vi "Controller FA File Management Loop.vi"(7 "Sync Objects":T1, 8 "error in (no error)":errorcluster, 11 "FOFB Configuration":T5={"FOFB Parameters"={"Network"={"FOFB Controller IP"="", "LNLS Control Network IP"="", "LNLS Control Network Power Supplies TCP Port"=0, "LNLS Control Network FOFB Configuration TCP Port"=0, "Data Server TCP Port"=0, "Monitoring Data TCP Port"=0, "Configuration GUI TCP Port"=0, "TCP Listening Timeout"=0}, "Fast Acquisition"={"Acquisition Period"=0, "Data Buffer Size"=0}, "Response Matrix Measurement"={"Step Amplitude"=0.0, "Time Between Steps"=0, "Step Duration"=0, "Number of Averages"=0}, "Correction Algorithm"={"Correction Period"=0, "Reference Orbit Path"=path "", "Response Matrix Path"=path "", "Correction Matrix Path"=path "", "Horizontal Correction Factor"=0.0, "Vertical Correction Factor"=0.0, "Beam Current FOFB Threshold"=0.0, "Decouple H-V"=FALSE}, "Acquisition Network"=[], "Actuation Network"=[]}, "Number of Acquisition Chassis"=0, "Number of Actuation Chassis"=0, "Number of BPM Readings"=0, "BPM Reading Names"=[], "Selected BPM Readings"=[0, 1, 2, 3, 4, 5, 6, 7, 8, 9, 10, 11, 12, 13, 14, 15, 16, 17, 18, 19, 20, 21, 22, 23, 24, 25, 26, 27, 28, 29, 30, 31, 32, 33, 34, 35, 36, 37, 38, 39, 40, 41, 42, 43, 44, 45, 46, 47, 48, 49], "Number of Correctors"=0, "Corrector Names"=[], "Selected Correctors"=[0, 1, 2, 3, 4, 5, 6, 7, 8, 9, 10, 11, 12, 13, 14, 15, 16, 17, 18, 19, 20, 21, 22, 23, 24, 25, 26, 27, 28, 29, 30, 31, 32, 33, 34, 35, 36, 37, 38, 39, 40, 41, 42, 43, 44, 45, 46, 47, 48, 49], "Reference Orbit"=[], "Response Matrix"=[], "Correction Matrix"=[], "Acquisition Chassis Names"=[], "Actuation Chassis Names"=[], "Acquisition Variables"=[], "Actuation Variables"=[], "PS Matrix Mapping"=[], "Inverse PS Matrix Mapping"=[], "Response Matrix Beam Energy (MeV)"=0.0, "PID Parameters"=[], "BPM Planes"=[], "Corrector Planes"=[], "RMM Step Factor"=[]}) -> (0 "error out":errorcluster)   [LabVIEW 2011, in "Controller VIs.lvlib"]
uses:
  Controller VIs.lvlib
  Types Definitions/Type FOFB Configuration.ctl
  Types Definitions/Type FOFB Parameters.ctl
  Types Definitions/Type Network Configuration.ctl
  Types Definitions/Type FA Configuration.ctl
  Types Definitions/Type Response Matrix Measurement Configuration.ctl
  Types Definitions/Type Correction Algorithm Configuration.ctl
  Types Definitions/Type Acquisition Network Configuration.ctl
  Types Definitions/Type Actuation Network Configuration.ctl
  Types Definitions/Type PID Parameters.ctl
  Types Definitions/Type Synchronization Objects.ctl
  Types Definitions/Type Blocking Synchronization Objects.ctl
  Types Definitions/Type FA Request Parameters.ctl
  Types Definitions/Type BPM and PS select cluster.ctl
  Types Definitions/Type FA File Parameters.ctl
  Types Definitions/Type Monitoring Data.ctl
  Types Definitions/Type Diagnostics Data.ctl
  Types Definitions/Type CPU Loads Array.ctl
  Types Definitions/Type CPU Loads.ctl
  Types Definitions/Type Non-blocking Synchronization Objects.ctl
  Types Definitions/Type FOFB Variables.ctl
  Types Definitions/Type Actuation State.ctl
  <vilib>/Platform/TimedLoop/XDataNode/timing_clust.ctl
  <vilib>/Platform/TimedLoop/XDataNode/nitl_modes.ctl
  <vilib>/Platform/TimedLoop/XDataNode/wakeup.ctl
  <vilib>/Platform/TimedLoop/XDataNode/XDataNode.xnode
  File VIs.lvlib
  Type Definitions.lvlib
  Common VIs.lvlib
  <vilib>/Platform/TimedLoop/XDataNode/XDNodeRunTimeDep.lvlib
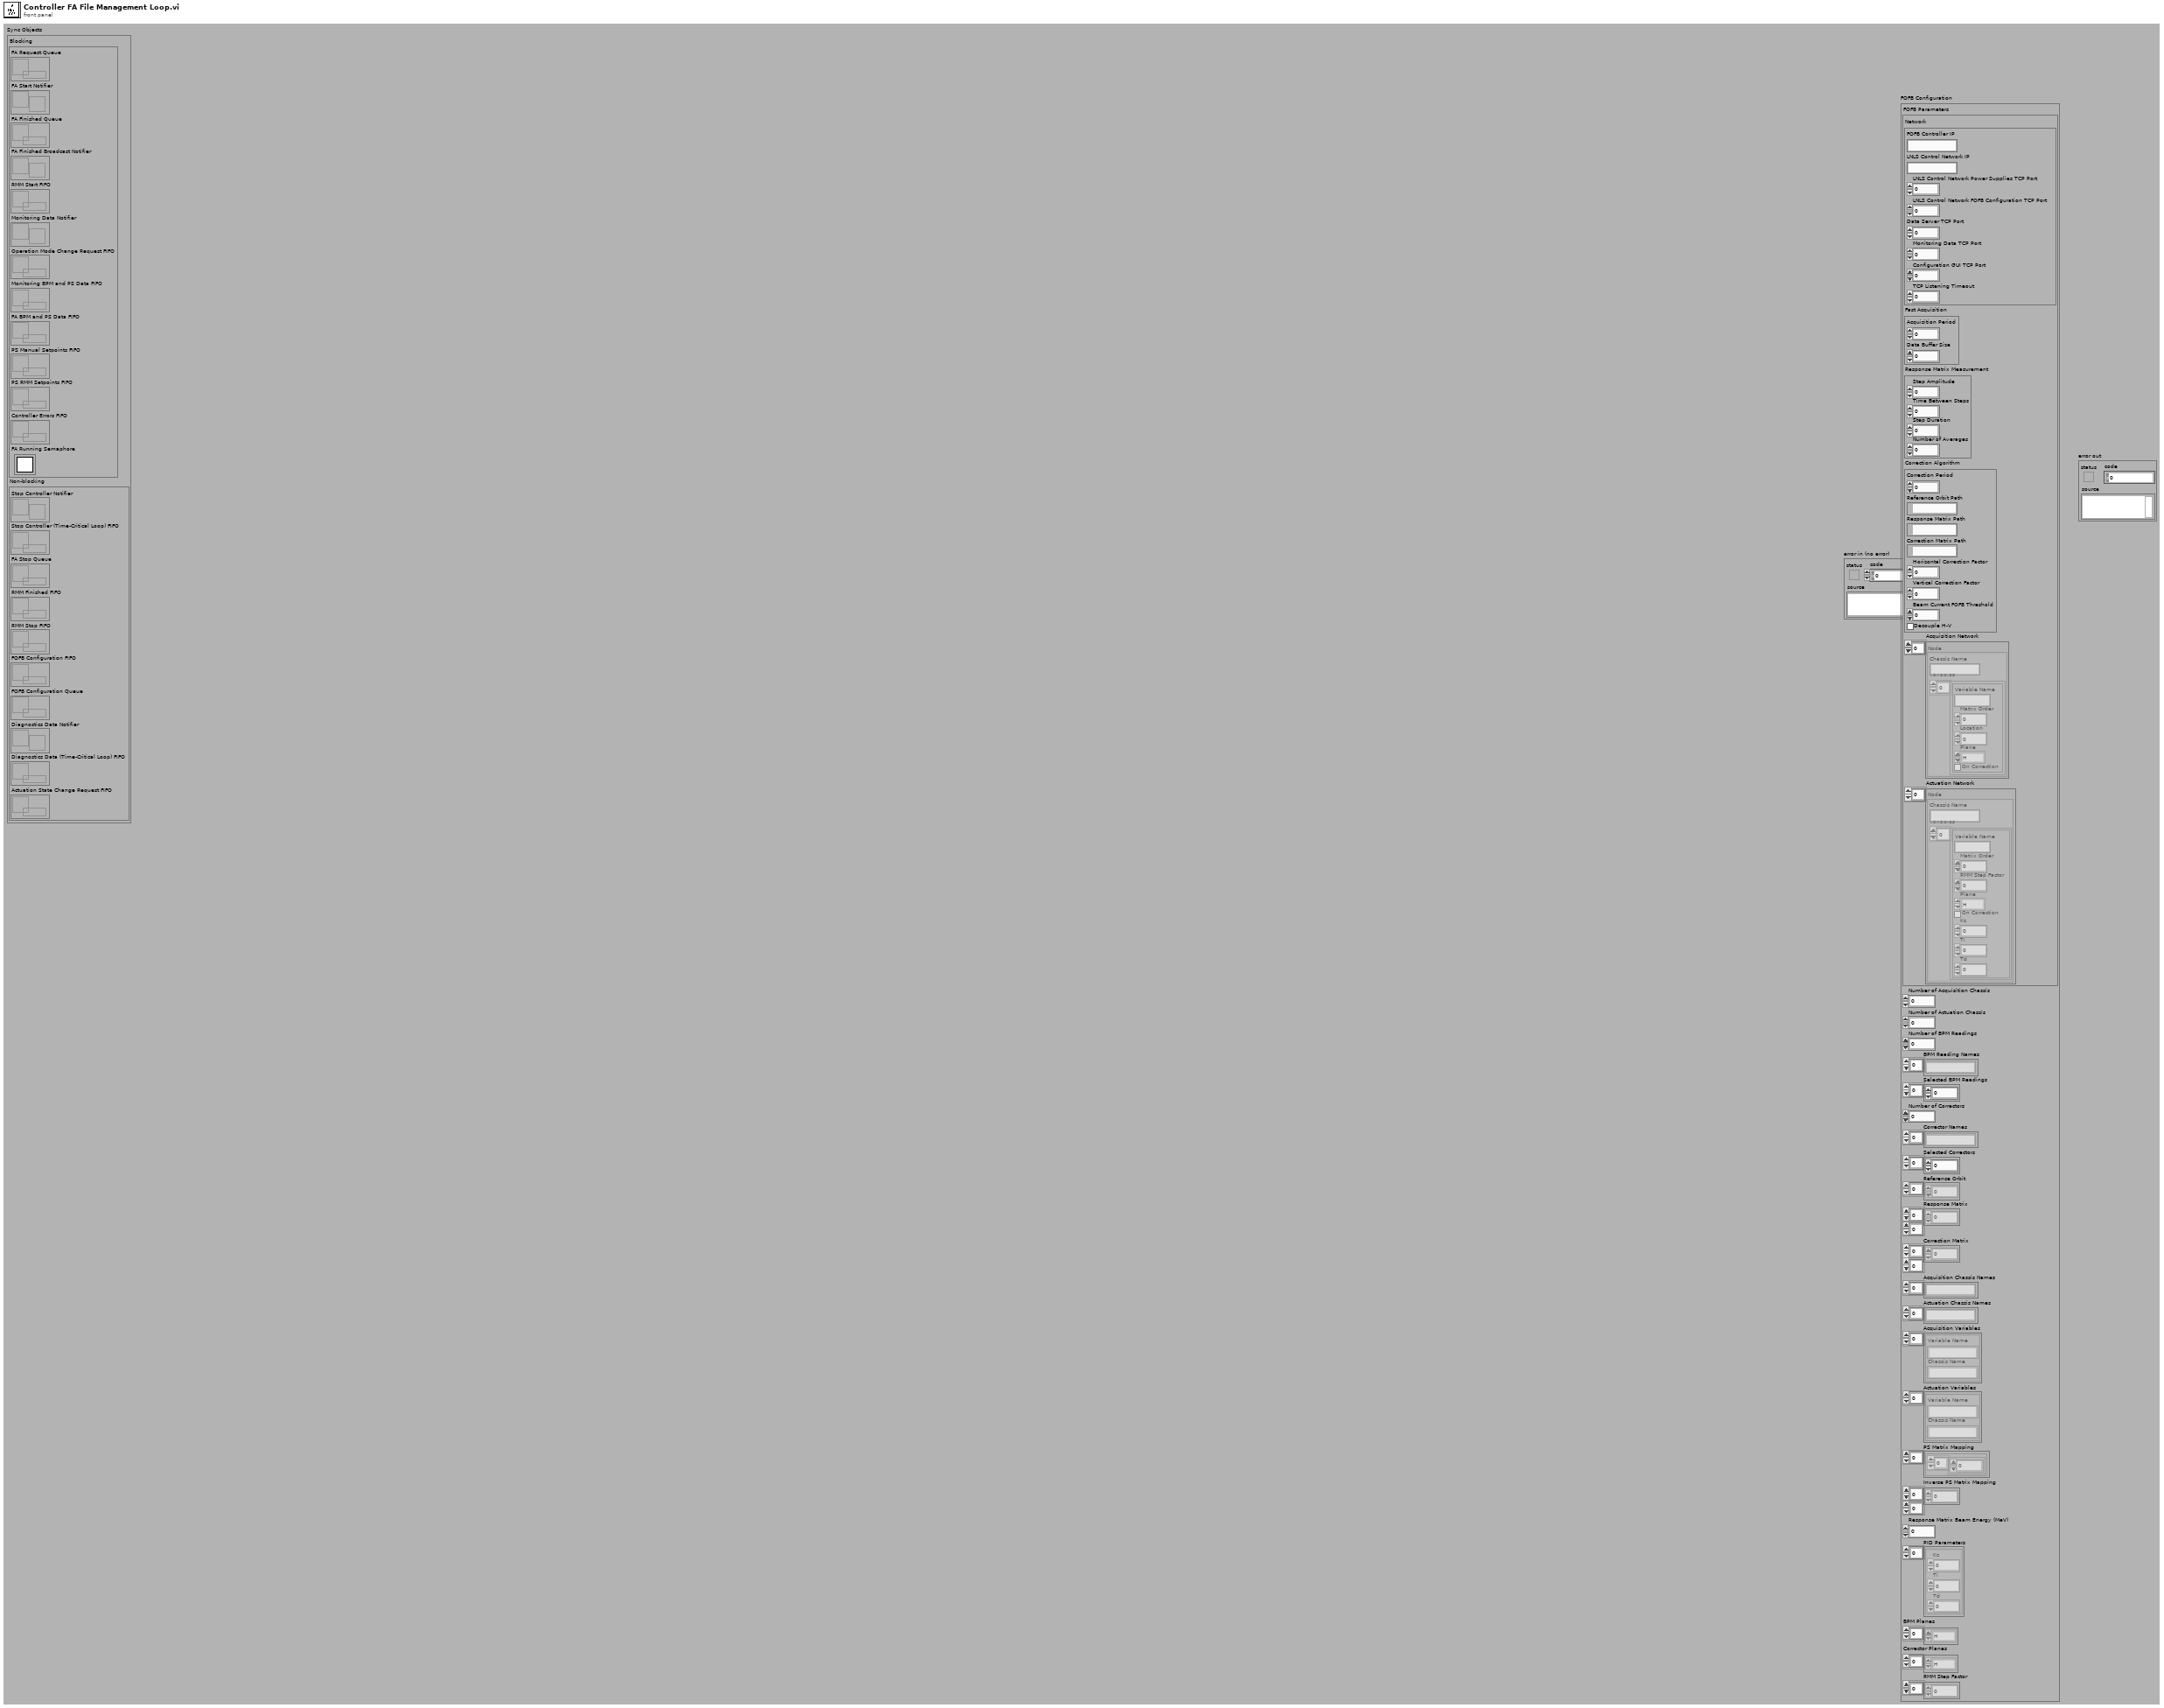
[diagram p1: front panel]
types:
  T1 = typedef "Type Definitions.lvlib/Type Synchronization Objects.ctl" = cluster{"Blocking":T2, "Non-blocking":T4}
  T2 = typedef "Type Definitions.lvlib/Type Blocking Synchronization Objects.ctl" = cluster{"FA Request Queue":refnum<queue>, "FA Start Notifier":refnum<notifier>, "FA Finished Queue":refnum<queue>, "FA Finished Broadcast Notifier":refnum<notifier>, "RMM Start FIFO":refnum<k33>, "Monitoring Data Notifier":refnum<notifier>, "Operation Mode Change Request FIFO":refnum<k33>, "Monitoring BPM and PS Data FIFO":refnum<k33>, "FA BPM and PS Data FIFO":refnum<k33>, "PS Manual Setpoints FIFO":refnum<k33>, "PS RMM Setpoints FIFO":refnum<k33>, "Controller Errors FIFO":refnum<k33>, "FA Running Semaphore":T3}
  T3 = typedef "Semaphore RefNum" = refnum<k1>
  T4 = typedef "Type Definitions.lvlib/Type Non-blocking Synchronization Objects.ctl" = cluster{"Stop Controller Notifier":refnum<notifier>, "Stop Controller (Time-Critical Loop) FIFO":refnum<k33>, "FA Stop Queue":refnum<queue>, "RMM Finished FIFO":refnum<k33>, "RMM Stop FIFO":refnum<k33>, "FOFB Configuration FIFO":refnum<k33>, "FOFB Configuration Queue":refnum<queue>, "Diagnostics Data Notifier":refnum<notifier>, "Diagnostics Data (Time-Critical Loop) FIFO":refnum<k33>, "Actuation State Change Request FIFO":refnum<k33>}
  T5 = typedef "Type Definitions.lvlib/Type FOFB Configuration.ctl" = cluster{"FOFB Parameters":T6, "Number of Acquisition Chassis":i32, "Number of Actuation Chassis":i32, "Number of BPM Readings":i32, "BPM Reading Names":string[], "Selected BPM Readings":u32[], "Number of Correctors":i32, "Corrector Names":string[], "Selected Correctors":u32[], "Reference Orbit":dbl[], "Response Matrix":dbl[][], "Correction Matrix":dbl[][], "Acquisition Chassis Names":string[], "Actuation Chassis Names":string[], "Acquisition Variables":cluster{"Variable Name":string, "Chassis Name":string}[], "Actuation Variables":cluster{"Variable Name":string, "Chassis Name":string}[], "PS Matrix Mapping":cluster{u32[]}[], "Inverse PS Matrix Mapping":u32[][], "Response Matrix Beam Energy (MeV)":dbl, "PID Parameters":T13[], "BPM Planes":enum8{"H", "V"}[], "Corrector Planes":enum8{"H", "V"}[], "RMM Step Factor":dbl[]}
  T6 = typedef "Type Definitions.lvlib/Type FOFB Parameters.ctl" = cluster{"Network":T7, "Fast Acquisition":T8, "Response Matrix Measurement":T9, "Correction Algorithm":T10, "Acquisition Network":T11, "Actuation Network":T12}
  T7 = typedef "Type Definitions.lvlib/Type Network Configuration.ctl" = cluster{"FOFB Controller IP":string, "LNLS Control Network IP":string, "LNLS Control Network Power Supplies TCP Port":u16, "LNLS Control Network FOFB Configuration TCP Port":u16, "Data Server TCP Port":u16, "Monitoring Data TCP Port":u16, "Configuration GUI TCP Port":u16, "TCP Listening Timeout":i32}
  T8 = typedef "Type Definitions.lvlib/Type FA Configuration.ctl" = cluster{"Acquisition Period":u32, "Data Buffer Size":u32}
  T9 = typedef "Type Definitions.lvlib/Type Response Matrix Measurement Configuration.ctl" = cluster{"Step Amplitude":dbl, "Time Between Steps":u32, "Step Duration":u32, "Number of Averages":u32}
  T10 = typedef "Type Definitions.lvlib/Type Correction Algorithm Configuration.ctl" = cluster{"Correction Period":u32, "Reference Orbit Path":path, "Response Matrix Path":path, "Correction Matrix Path":path, "Horizontal Correction Factor":dbl, "Vertical Correction Factor":dbl, "Beam Current FOFB Threshold":dbl, "Decouple H-V":bool}
  T11 = typedef "Type Definitions.lvlib/Type Acquisition Network Configuration.ctl" = cluster{"Chassis Name":string, "Variables":cluster{"Variable Name":string, "Matrix Order":u32, "Location":dbl, "Plane":enum8{"H", "V"}, "On Correction":bool}[]}[]
  T12 = typedef "Type Definitions.lvlib/Type Actuation Network Configuration.ctl" = cluster{"Chassis Name":string, "Variables":cluster{"Variable Name":string, "Matrix Order":u32, "RMM Step Factor":dbl, "Plane":enum8{"H", "V"}, "On Correction":bool, "Kc":dbl, "Ti":dbl, "Td":dbl}[]}[]
  T13 = typedef "Type Definitions.lvlib/Type PID Parameters.ctl" = cluster{"Kc":fxp<+/-,16,8>, "Ti":fxp<+/-,16,8>, "Td":fxp<+/-,16,8>}
  T14 = typedef "XDNodeRunTimeDep.lvlib/timing_clust.ctl" = cluster{"Expected End [f-1]":u64, "Actual End [f-1]":u64, "Finished Late? [f-1]":bool, "Expected End [i-1]":u64, "Actual End [i-1]":u64, "Finished Late? [i-1]":bool, "Expected Start [i]":u64, "Actual Start [i]":u64, "Expected Start [f]":u64, "Actual Start [f]":u64, "Source Name":string, "Structure Name":string, "Period":i64, "Deadline":i64, "Offset":i64, "Start":i64, "Priority":i32, "Timeout":i32, "Mode":T15, "Wakeup Reason":T16, "Error":errorcluster, "Source Type":string, "Secondary Source Type":string, "Global End Time":u64, "Global Start Time":u64, "Frame Duration":u64, "Iteration Duration":u64, "Assigned CPU":i32, "I/O Scan Engine Mode":u32}
  T15 = typedef "XDNodeRunTimeDep.lvlib/nitl_modes.ctl" = enum32{"No Change", "Process missed periods, maintain original phase", "Discard missed periods, maintain original phase", "Process missed periods, ignore original phase", "Discard missed periods, ignore original phase"}
  T16 = typedef "XDNodeRunTimeDep.lvlib/wakeup.ctl" = enum32{"Normal", "Aborted", "Asynchronous wakeup", "Timing source error", "Timed loop error", "Timeout"}
  T17 = typedef "Type Definitions.lvlib/Type FA File Parameters.ctl" = cluster{"FA Parameters":T18, "File Reference":refnum<file>}
  T18 = typedef "Type Definitions.lvlib/Type FA Request Parameters.ctl" = cluster{"Number of Samples":u32, "BPM and PS Selection":T19, "Filename":string}
  T19 = typedef "Type Definitions.lvlib/Type BPM and PS select cluster.ctl" = cluster{"BPM index array":u32[], "PS index array ":u32[]}
  T20 = enum16{"open", "replace", "create", "open or create", "replace or create", "replace or create with confirmation"}
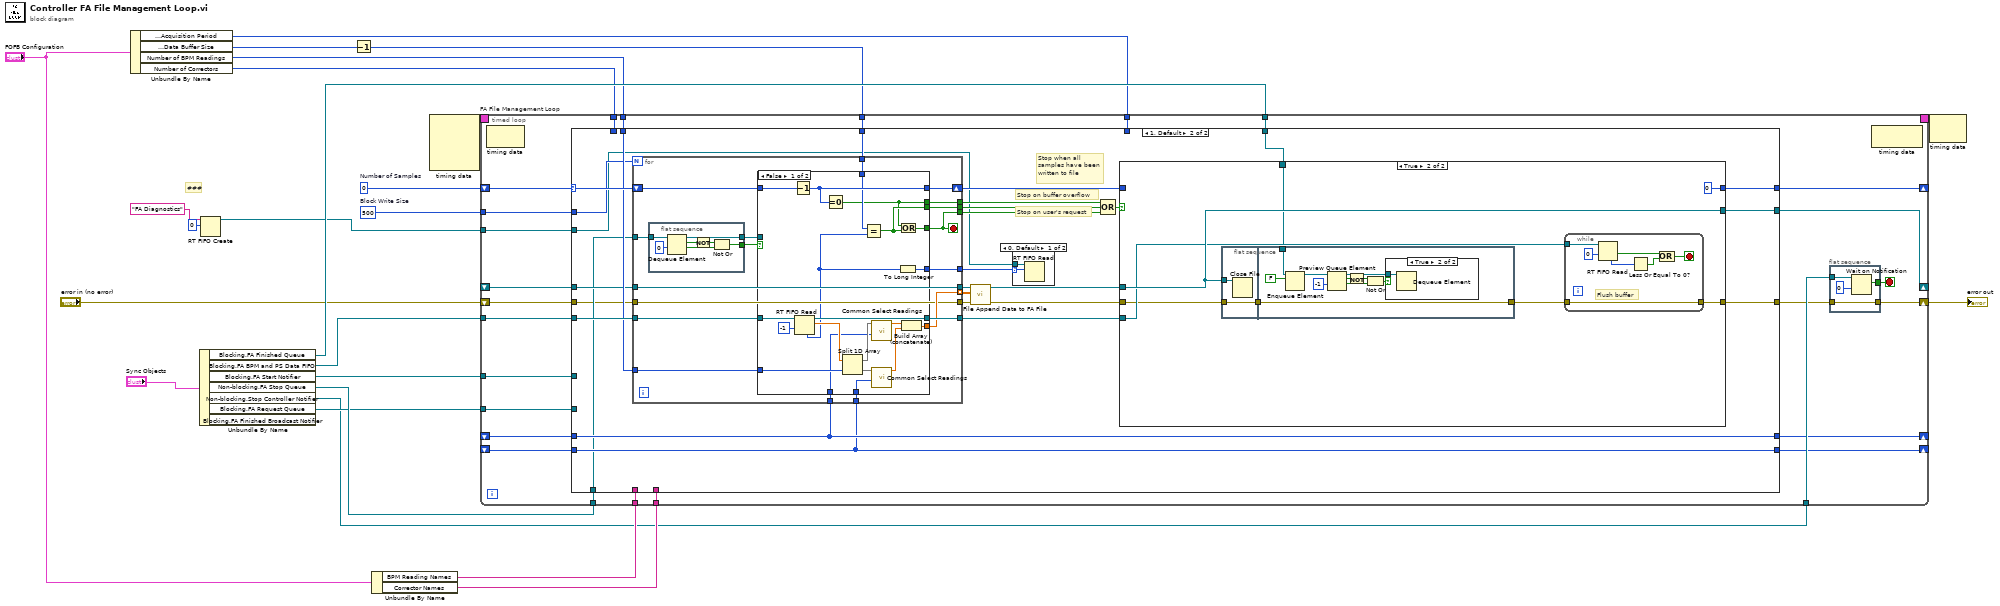
[diagram p0: block diagram]
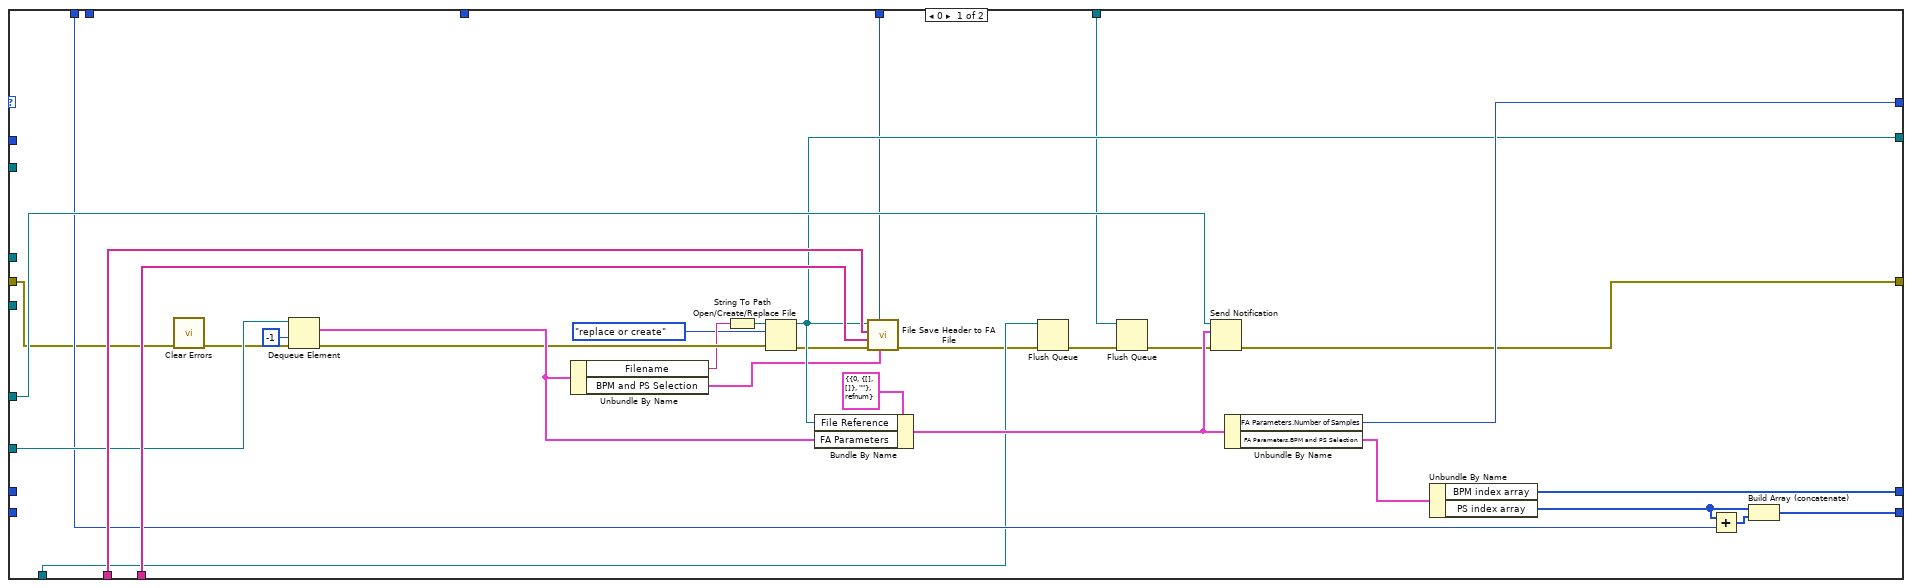
[diagram p2: hidden frame]
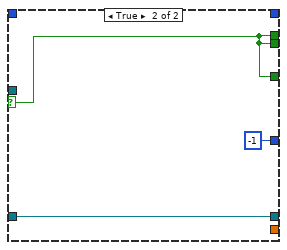
[diagram p4: hidden frame]
diagram:
  w7 = 500  # Block Write Size
  w22 = u32 0  # Number of Samples
  # "###"
  n1 = Unbundle By Name("FOFB Configuration") -> ("FOFB Parameters.Fast Acquisition.Acquisition Period"=w6:u32, "FOFB Parameters.Fast Acquisition.Data Buffer Size"=w20:u32, "Number of BPM Readings"=w9:i32, "Number of Correctors"=w8:i32)
  n2 = Unbundle By Name("Sync Objects") -> ("Blocking.FA Finished Queue"=w21:refnum<queue>, "Blocking.FA BPM and PS Data FIFO"=w23:refnum<k33>, "Blocking.FA Start Notifier"=w13:refnum<notifier>, "Non-blocking.FA Stop Queue"=w19:refnum<queue>, "Non-blocking.Stop Controller Notifier"=w12:refnum<notifier>, "Blocking.FA Request Queue"=w14:refnum<queue>)  [unwired: 1 out]
  n3 = RT FIFO Create(0:"FA Diagnostics" ("name (unnamed)"), 1:0 ("# elements")) -> (8:w1:refnum<k33>)  [unwired: 6 in, 2 out]
  n4 = Decrement(x=w20) -> (x-1=w10:u32)
  n5 = Unbundle By Name("FOFB Configuration") -> ("BPM Reading Names"=w16:string[], "Corrector Names"=w15:string[])
  n6 = node-c288() -> (w5:T14)  [unwired: 4 in]
  n7 = timed-loop "FA File Management Loop" {
    shift-right: [w39] -> w11
    shift-left: "error in (no error)" -> [w50]
    shift-right: [w42] -> _
    shift-left: w22 -> [w48]
    shift-right: [w49] -> _
    shift-left: _ -> [w47]
    tunnel: w13 -> [w46]
    tunnel: w23 -> [w45]
    tunnel: w12 -> [w44]
    tunnel: w19 -> [w41]
    tunnel: w21 -> [w40]
    tunnel: w9 -> [w38]
    tunnel: w8 -> [w36]
    tunnel: w16 -> [w35]
    tunnel: w15 -> [w34]
    tunnel: w14 -> [w33]
    shift-right: [w31] -> _
    shift-left: _ -> [w29]
    shift-right: [w32] -> _
    shift-left: _ -> [w30]
    tunnel: w10 -> [w28]
    tunnel: w7 -> [w27]
    tunnel: w6 -> [w26]
    timing: w5 -> [_]
    timing-out: [_] -> w4
    tunnel: w1 -> [w25]
    stop <- w43 stop-if-true
    n8 = node-c288() -> ()  [unwired: 1 in, 1 out]
    n9 = case shown="1, Default" w48 {
      selector: w48 -> [_ w113]
      tunnel: w50 -> [w64 w91]
      tunnel: [w81 w109] -> w49
      tunnel: [w87 w110] -> w42
      tunnel: [w82 w108] -> w37
      tunnel: w47 -> [_ w99]
      tunnel: w46 -> [w83 _]
      tunnel: w45 -> [_ w114]
      tunnel: w41 -> [w59 w92]
      tunnel: w40 -> [w60 w111]
      tunnel: w38 -> [_ w107]
      tunnel: w36 -> [w78 _]
      tunnel: w35 -> [w86 _]
      tunnel: w34 -> [w85 _]
      tunnel: w33 -> [w84 _]
      tunnel: [w80 w105] -> w32
      tunnel: [w79 w104] -> w31
      tunnel: w30 -> [_ w105]
      tunnel: w29 -> [_ w104]
      tunnel: w28 -> [_ w101]
      tunnel: w27 -> [_ w98]
      tunnel: w26 -> [w66 _]
      tunnel: w25 -> [_ w89]
      frame 0 {
        n10 = call <vilib>:"Clear Errors.vi"("error in (no error)"=w64) -> ("error out"=w65:errorcluster)  [unwired: 6 in]
        n11 = Dequeue Element(queue=w84, timeout in ms (-1)=-1, error in (no error)=w65) -> (element=w77:T18, error out=w76:errorcluster)  [unwired: 2 out]
        n12 = Unbundle By Name(w77) -> ("Filename"=w75:string, "BPM and PS Selection"=w71:T19)
        n13 = String To Path(string=w75) -> (path=w74:path)
        n14 = Open/Create/Replace File(file path (use dialog)=w74, error in=w76, operation (0:open)=T20."replace or create") -> (refnum out=w81:refnum<file>, error out=w72:errorcluster)  [unwired: 3 in, 1 out]
        n15 = Bundle By Name(cluster=T17 {"FA Parameters"={"Number of Samples"=0, "BPM and PS Selection"={"BPM index array"=[], "PS index array "=[]}, "Filename"=""}, "File Reference"=refnum} ("File Parameters"), "File Reference"=w81, "FA Parameters"=w77) -> (w63:T17)
        n16 = call "File Save Header to FA File.vi"("BPM and PS selection"=w71, "Acquisition period (us)"=w66, "error in (no error)"=w72, "PS Reading Names"=w85, "BPM Reading Names"=w86, "FA File Reference"=w81) -> ("error out"=w58:errorcluster)  [unwired: 5 in]
        n17 = Flush Queue(queue=w59, error in (no error)=w58) -> (error out=w57:errorcluster)  [unwired: 2 out]
        n18 = Flush Queue(queue=w60, error in (no error)=w57) -> (error out=w61:errorcluster)  [unwired: 2 out]
        n19 = Send Notification(notification=w63, notifier=w83, error in (no error)=w61) -> (error out=w82:errorcluster)  [unwired: 1 out]
        n20 = Unbundle By Name(w63) -> ("FA Parameters.Number of Samples"=w87:u32, "FA Parameters.BPM and PS Selection"=w67:T19)
        n21 = Unbundle By Name(w67) -> ("BPM index array"=w80:u32[], "PS index array"=w68:u32[])
        n22 = Add(x=w68, y=w78) -> (x+y=w69:u32[])
        n23 = Build Array (concatenate)(w68, w69) -> (w79:u32[])
      }
      frame 1, Default {
        # "Stop on user's request"
        # "Stop on buffer overflow"
        # "Stop when all\nsamples have been\nwritten to file"
        n24 = for {
          N: w98 -> [_]
          tunnel: w114 -> [w134]
          tunnel: [w132] -> w112
          tunnel: w107 -> [w131]
          tunnel: w105 -> [w130]
          tunnel: w104 -> [w129]
          tunnel: [w125] -> w103
          tunnel: w101 -> [w127]
          tunnel: [w126] -> w100
          tunnel: w91 -> [w121]
          tunnel: [w121] -> w95
          tunnel: w99 -> [w124]
          tunnel: [w124] -> w94
          tunnel: [w123] -> w93 mode=indexing
          shift-right: [w128] -> w102
          shift-left: w113 -> [w133]
          tunnel: w92 -> [w122]
          tunnel: [w119] -> w90
          tunnel: [w118] -> w88
          stop <- w119 stop-if-true
          n25 = flat-sequence {
            tunnel: w122 -> [w141]
            tunnel: [w137] -> w120
            tunnel: [w139] -> w117
            frame #0 {
              n26 = Dequeue Element(queue=w141, timeout in ms (-1)=0) -> (queue out=w139:refnum<queue>, element=w136:bool, timed out?=w135:bool)  [unwired: 1 in, 1 out]
              n27 = Not(x=w136) -> (.not. x?=w138:bool)
              n28 = Not Or(1:w135, 2:w138) -> (0:w137:bool)
            }
          }
          n29 = case shown="False" w120 {
            selector: w120 -> [_ w162]
            tunnel: w134 -> [w161 w164]
            tunnel: w133 -> [w160 _]
            tunnel: [w159 w164] -> w132
            tunnel: w131 -> [w158 _]
            tunnel: w130 -> [w151 _]
            tunnel: w129 -> [w150 _]
            tunnel: [w149 _] -> w128
            tunnel: w127 -> [w148 _]
            tunnel: [w147 w162] -> w126
            tunnel: [w146 w162] -> w125
            tunnel: [w145 w162] -> w119
            tunnel: [w144 _] -> w123
            tunnel: [w143 -1 ("# elements")] -> w118
            tunnel: w117 -> [_ _]
            frame False {
              n30 = Decrement(x=w160) -> (x-1=w149:u32)
              n31 = RT FIFO Read(0:w161, 2:-1 ("timeout in ms (0)")) -> (7:w142:u32, 8:w159:refnum<k33>, 9:w156:dbl[])  [unwired: 2 in, 2 out]
              n32 = Equal To 0?(x=w149) -> (x = 0?=w146:bool)
              n33 = Split 1D Array(array=w156, index=w158) -> (first subarray=w153:dbl[], second subarray=w155:dbl[])
              n34 = Equal?(x=w148, y=w142) -> (x = y?=w147:bool)
              n35 = call "Common Select Readings.vi"("Selected Readings"=w151, "Readings"=w153) -> ("Readings Subset"=w152:dbl[])  [unwired: 9 in]
              n36 = call "Common Select Readings.vi"("Selected Readings"=w150, "Readings"=w155) -> ("Readings Subset"=w154:dbl[])  [unwired: 9 in]
              n37 = To Long Integer(number=w142) -> (32bit integer=w143:i32)
              n38 = Or(x=w146, y=w147) -> (x .or. y?=w145:bool)
              n39 = Build Array (concatenate)(w152, w154) -> (w144:dbl[])
            }
            frame True {
            }
          }
        }
        n40 = call "File Append Data to FA File.vi"("error in (no error)"=w95, "Data"=w93, "FA File Reference"=w94) -> ("error out"=w96:errorcluster, "FA File Reference"=w97:refnum<file>)  [unwired: 6 in]
        n41 = case shown="0, Default" w88 {
          selector: w88 -> [w115 _]
          tunnel: w89 -> [w116 _]
          frame 0, Default {
            n42 = RT FIFO Read(0:w116, 1:w115) -> ()  [unwired: 2 in, 5 out]
          }
          frame -1 {
          }
        }
        n43 = Compound Arithmetic op=OR(w103, w100, w90) -> (w106:bool)
        n44 = case shown="True" w106 {
          tunnel: w102 -> [w166 _]
          tunnel: w112 -> [_ w173]
          tunnel: w97 -> [w167 w174]
          tunnel: [w166 u32 0] -> w110
          tunnel: [w167 w174] -> w109
          tunnel: [w165 w170] -> w108
          tunnel: w96 -> [w165 w172]
          tunnel: w111 -> [_ w168]
          frame False {
          }
          frame True {
            n45 = flat-sequence {
              tunnel: w174 -> [w184]
              tunnel: w172 -> [w183]
              tunnel: [w183] -> w169
              tunnel: [w194] -> w171
              tunnel: w169 -> [w194]
              tunnel: w168 -> [w185]
              frame #0 {
                n46 = Close File(refnum=w184) -> ()  [unwired: 1 in, 2 out]
              }
              frame #1 {
                n47 = Enqueue Element(queue=w185, element=FALSE ("notification")) -> (queue out=w186:refnum<queue>)  [unwired: 2 in, 2 out]
                n48 = Preview Queue Element(queue=w186, timeout in ms (-1)=-1) -> (queue out=w191:refnum<queue>, element=w189:bool, timed out?=w192:bool)  [unwired: 1 in, 1 out]
                n49 = Not(x=w189) -> (.not. x?=w188:bool)
                n50 = Not Or(1:w192, 2:w188) -> (0:w193:bool)
                n51 = case shown="True" w193 {
                  tunnel: w191 -> [_ w195]
                  frame False {
                  }
                  frame True {
                    n52 = Dequeue Element(queue=w195) -> ()  [unwired: 2 in, 4 out]
                  }
                }
              }
            }
            n53 = while {
              tunnel: w173 -> [w177]
              tunnel: [w176] -> w170
              tunnel: w171 -> [w176]
              stop <- w178 stop-if-true
              # "Flush buffer"
              n54 = RT FIFO Read(0:w177, 2:0 ("timeout in ms (0)")) -> (7:w180:u32, 10:w181:bool)  [unwired: 2 in, 3 out]
              n55 = Less Or Equal To 0?(x=w180) -> (x <= 0?=w179:bool)
              n56 = Compound Arithmetic op=OR(w181, w179) -> (w178:bool)
            }
          }
        }
      }
    }
    n57 = flat-sequence {
      tunnel: w44 -> [w55]
      tunnel: [w54] -> w43
      tunnel: w37 -> [w53]
      tunnel: [w53] -> w39
      frame #0 {
        n58 = Wait on Notification(notifier=w55, timeout in ms (-1)=0) -> (notification=w54:bool)  [unwired: 2 in, 3 out]
      }
    }
    n59 = node-c288() -> ()  [unwired: 1 in, 1 out]
  }
  "error out" <- w11
  n60 = node-c288(w4) -> ()  [unwired: 1 out]
